vi "Measure vs B2DvsGatesweep.vi"() -> ()   [LabVIEW 2009]
doc: "This VI is an example operator panel.\n\nThe VI contains a table for the field values that may be configured manually, or loaded by checking the \"Prompt for File\" box. The data file should contain 3 columns of data, with each column delimited by a tab character.\n\nBefore the VI is executed, set the desired field units and coordinate system. Once the VI is started, follow the directions in the STATUS indicator to operate. Once a field value is achieved, it will be held indefinitely with no user intervention.\n\nThe present field is displayed in the selected units and coordinate system. The present field is queried once per second.\n\nIf a field point is specified that is outside the limits for the magnet, the VI will abort execution."
uses:
  <vilib>/Utility/file.llb/Read From Spreadsheet File (DBL).vi
panel:
  out "HP":T1(graph)={"measured data"=[130.77697934473076, 131.17238359064999, 131.57493282279165, 131.97089096284472, 132.3709005627829, 132.7747269835502, 133.17115299337118, 133.57699453159358, 133.97291907281786, 134.37163450772164, 134.7728190578919, 135.17563033959266, 135.57333372461295, 135.97830344291987, 136.37202071047088, 136.77617688548457, 137.17728611854096, 137.57344246367185, 137.96927398938195, 138.37484712631183, 138.7678966828463, 139.1744152195974, 139.5694101008014, 139.9620548045032, 140.3756352936819, 140.76443013035026, 141.1688823561444, 141.56815184223575, 141.9675976417151, 142.3659953584458, 142.775676716873, 143.16379154430956, 143.57809589273134, 143.96940395419173, 144.37063731617485, 144.76393855420042, 145.16100725100878, 145.5613313376955, 145.9608116195239, 146.37481274459287, 146.76791709360782, 147.16896149127172, 147.5663143604346, 147.9678028289989, 148.36962760092925, 148.76598884997566, 149.16767338072717, 149.56607764958403, 149.95999407346423, 150.3722468362733, 150.76361618206533, 151.15525055318153, 151.57358356130908, 151.9672547235955, 152.360163563412, 152.76137159791082, 153.15948892689605, 153.56793804327447, 153.9626908891637, 154.35791457944399, 154.76495537165297, 155.1633906497064, 155.56156935652382, 155.96111561211768, 156.36610319740612, 156.76559958179956, 157.17093878264262, 157.56689125105595, 157.96437052200662, 158.376205209266, 158.76161261329872, 159.16724590816438, 159.55971274891448, 159.96783078495864, 160.36059978391282, 160.75915896709176, 161.17541940848784, 161.56387349300712, 161.96414973052572, 162.36209894569686], "measured data"=[47.8127675, 47.3142275, 46.9315925, 46.6304225, 46.0396825, 45.6777125, 45.4570175, 45.070972499999996, 44.789265, 44.3558025, 43.6591325, 43.409885, 43.162465, 42.71473, 42.531679999999994, 42.226214999999996, 41.899212500000004, 41.3661625, 41.03545, 40.637135, 40.367885, 40.046705, 39.865300000000005, 39.57427, 39.035422499999996, 38.758669999999995, 38.5814575, 38.362825, 37.764005, 37.63395250000001, 37.1175925, 15.572479999999999, -4.558832499999999, -4.02452, 18.98894, -4.1475925, -5.032675, 25.0248675, 27.1825925, 28.551062500000004, 27.772665, 26.5350725, 23.5985575, 27.104, 24.8567975, 23.797494999999998, 25.486569999999997, 24.9155175, 26.26794, 24.482997499999996, 25.039457499999997, 13.34384, 13.3442075, 13.3447275, 13.34462, 13.344155, 54.256817500000004, 13.3434, 13.3445175, 13.343632500000002, 13.3429575, 13.343734999999999, 13.3441525, -7.896862499999999, 13.344205, -8.8820475, 13.343815, 13.3419875, -24.604432499999998, 13.342722499999999, -6.686962499999998, 13.34337, 13.343815, 13.344335000000001, -23.786430000000003, 13.34392, 13.343657499999999, 13.3431125, 13.3426425, 13.342744999999999]}
  in  "go to zero at end of measurement":bool=TRUE
  out "fieldvalues":string[](array[string])=["0.5", "91"]
  out "LI":T1(graph)={"measured data"=[130.77697934473076, 131.17238359064999, 131.57493282279165, 131.97089096284472, 132.3709005627829, 132.7747269835502, 133.17115299337118, 133.57699453159358, 133.97291907281786, 134.37163450772164, 134.7728190578919, 135.17563033959266, 135.57333372461295, 135.97830344291987, 136.37202071047088, 136.77617688548457, 137.17728611854096, 137.57344246367185, 137.96927398938195, 138.37484712631183, 138.7678966828463, 139.1744152195974, 139.5694101008014, 139.9620548045032, 140.3756352936819, 140.76443013035026, 141.1688823561444, 141.56815184223575, 141.9675976417151, 142.3659953584458, 142.775676716873, 143.16379154430956, 143.57809589273134, 143.96940395419173, 144.37063731617485, 144.76393855420042, 145.16100725100878, 145.5613313376955, 145.9608116195239, 146.37481274459287, 146.76791709360782, 147.16896149127172, 147.5663143604346, 147.9678028289989, 148.36962760092925, 148.76598884997566, 149.16767338072717, 149.56607764958403, 149.95999407346423, 150.3722468362733, 150.76361618206533, 151.15525055318153, 151.57358356130908, 151.9672547235955, 152.360163563412, 152.76137159791082, 153.15948892689605, 153.56793804327447, 153.9626908891637, 154.35791457944399, 154.76495537165297, 155.1633906497064, 155.56156935652382, 155.96111561211768, 156.36610319740612, 156.76559958179956, 157.17093878264262, 157.56689125105595, 157.96437052200662, 158.376205209266, 158.76161261329872, 159.16724590816438, 159.55971274891448, 159.96783078495864, 160.36059978391282, 160.75915896709176, 161.17541940848784, 161.56387349300712, 161.96414973052572, 162.36209894569686], "measured data"=[47.8127675, 47.3142275, 46.9315925, 46.6304225, 46.0396825, 45.6777125, 45.4570175, 45.070972499999996, 44.789265, 44.3558025, 43.6591325, 43.409885, 43.162465, 42.71473, 42.531679999999994, 42.226214999999996, 41.899212500000004, 41.3661625, 41.03545, 40.637135, 40.367885, 40.046705, 39.865300000000005, 39.57427, 39.035422499999996, 38.758669999999995, 38.5814575, 38.362825, 37.764005, 37.63395250000001, 37.1175925, 15.572479999999999, -4.558832499999999, -4.02452, 18.98894, -4.1475925, -5.032675, 25.0248675, 27.1825925, 28.551062500000004, 27.772665, 26.5350725, 23.5985575, 27.104, 24.8567975, 23.797494999999998, 25.486569999999997, 24.9155175, 26.26794, 24.482997499999996, 25.039457499999997, 13.34384, 13.3442075, 13.3447275, 13.34462, 13.344155, 54.256817500000004, 13.3434, 13.3445175, 13.343632500000002, 13.3429575, 13.343734999999999, 13.3441525, -7.896862499999999, 13.344205, -8.8820475, 13.343815, 13.3419875, -24.604432499999998, 13.342722499999999, -6.686962499999998, 13.34337, 13.343815, 13.344335000000001, -23.786430000000003, 13.34392, 13.343657499999999, 13.3431125, 13.3426425, 13.342744999999999]}
  in  "Wait between \nVectors":bool=TRUE
  in  "PID Off":bool
  in  "Wait between \nVectors (ms)":u32=4000
  out "measured data":dbl[][](array[numeric])
  in  "Notes:":string="Datum: 6.04.12, Uhrzeit: 12:30,  T 4K,Winkelsweep 1° Winkelschritte, warten bei jedem Feldpunkt (measurevsB2Dv9.vi))4s, vectorsm1.txt, praktikumsprobenstab, Sweep  0.15, CrB auf CuBe Sensoren" caption="Notizen:"
  in  "Measurement File":path=path "D:/UserData/Matthias/Messungen/STO_LAOR124aufCantilever/120523/120523_R124_Gatevst"
  in  "Sample name:":string="CrB"
  in  "HP 1":bool=TRUE
  in  "GPIB HP":string="13"
  in  "LI 1":bool
  in  "GPIB L 1":string="8"
  out "Number of lines":i32=2
  in  "Operation":u16(ring)=1 items=["Stepwise", "Continous"]
  out "Ramp Rate along Vector (T/min)":dbl=0.15 format="%.3f"
  out "Current Ramp Rate Z (T/min)":dbl=0.015702717677741673 format="%.3f"
  out "Current Ramp Rate Y (T/min)":dbl=0.1491758179382072 format="%.3f"
  in  "User defined Ramp Rate (T/min)":bool=TRUE
  in  "User defined Ramp Rate (T/min)":dbl=0.5 format="%.3f"
  in  "Z-Axis Communications Config":T2={"GPIB address"=22, "GPIB bus"=1, "connection ID"=refnum, "IP"="111.111.111.1", "Active Comm Interface"=0, "Serial Port"="", "Programmer Type"=0} {"Programmer Type" items=["Model 430", "Model 420"]; "Active Comm Interface" items=["TCP/IP (Model 430 Only)", "RS232", "IEEE488"]}
  in  "Max Ramp Rate - Y Axis (A/s)":dbl=0.055 format="%.3f"
  in  "Max Ramp Rate - Z Axis (A/s)":dbl=0.19 format="%.3f"
  in  "Magnitude Limit (kG)":dbl=45.1 format="%.3f"
  in  "Y-Axis Communications Config":T2={"GPIB address"=22, "GPIB bus"=1, "connection ID"=refnum, "IP"="111.111.111.2", "Active Comm Interface"=0, "Serial Port"="", "Programmer Type"=0} {"Programmer Type" items=["Model 430", "Model 420"]; "Active Comm Interface" items=["TCP/IP (Model 430 Only)", "RS232", "IEEE488"]}
  out "Cartesian Display (T)":T3={"Y-Axis Field (T)"=0.01746, "Z-Axis Field (T)"=0.99986} {"Z-Axis Field (T)" format="%.3f"; "Y-Axis Field (T)" format="%.3f"}
  in  "Starting index":i32=1
  in  "Normal color":u32(colorbox)=11711154
  in  "Highlight color":u32(colorbox)=16711680
  in  "Prompt for File?":bool
  out "Continue Execution?":bool=TRUE
  out "error out":T4
  in  "error in":T4
  out "STATUS":string="Ramping to field vector 1..."
  in  "Ramping Control":u16(ring)=1 items=["NEXT VECTOR", "RAMPING", "HOLDING", "PAUSE", "ZERO"]
  out "Cartesian Display (kG)":T5 {"Z-Axis Field (kG)" format="%.3f"; "Y-Axis Field (kG)" format="%.3f"}
  in  "Field Values":string[][](table)=[["0", "1"], ["0", "0.5"]]
  out "Switch Heaters":bool=TRUE
  out "Polar Display (T)":T6={"q (degrees)"=89.97708168941708, "Field Magnitude (T)"=0.5000000399999984} {"Field Magnitude (T)" format="%.3f"; "q (degrees)" format="%.3f"}
  out "Polar Display (kG)":T7 {"Field Magnitude (kG)" format="%.3f"; "q (degrees)" format="%.3f"}
  in  "Coordinate System":u16(ring) items=["Cartesian", "Polar"]
  in  "Magnetic Field Units":u16(ring)=1 items=["kG", "Tesla"]
  # "Punkt für Punkt Messung, gotozero am Ende der Messung und switch heater off"
  # "Measurement Display"
  # "Measurement Settings"
  # "Magnet Settings"
  # "Max Ramp Rate z: 1.27 T/min\nMax Ramp Rate y: 0.17 T/min"
  # "Devices"
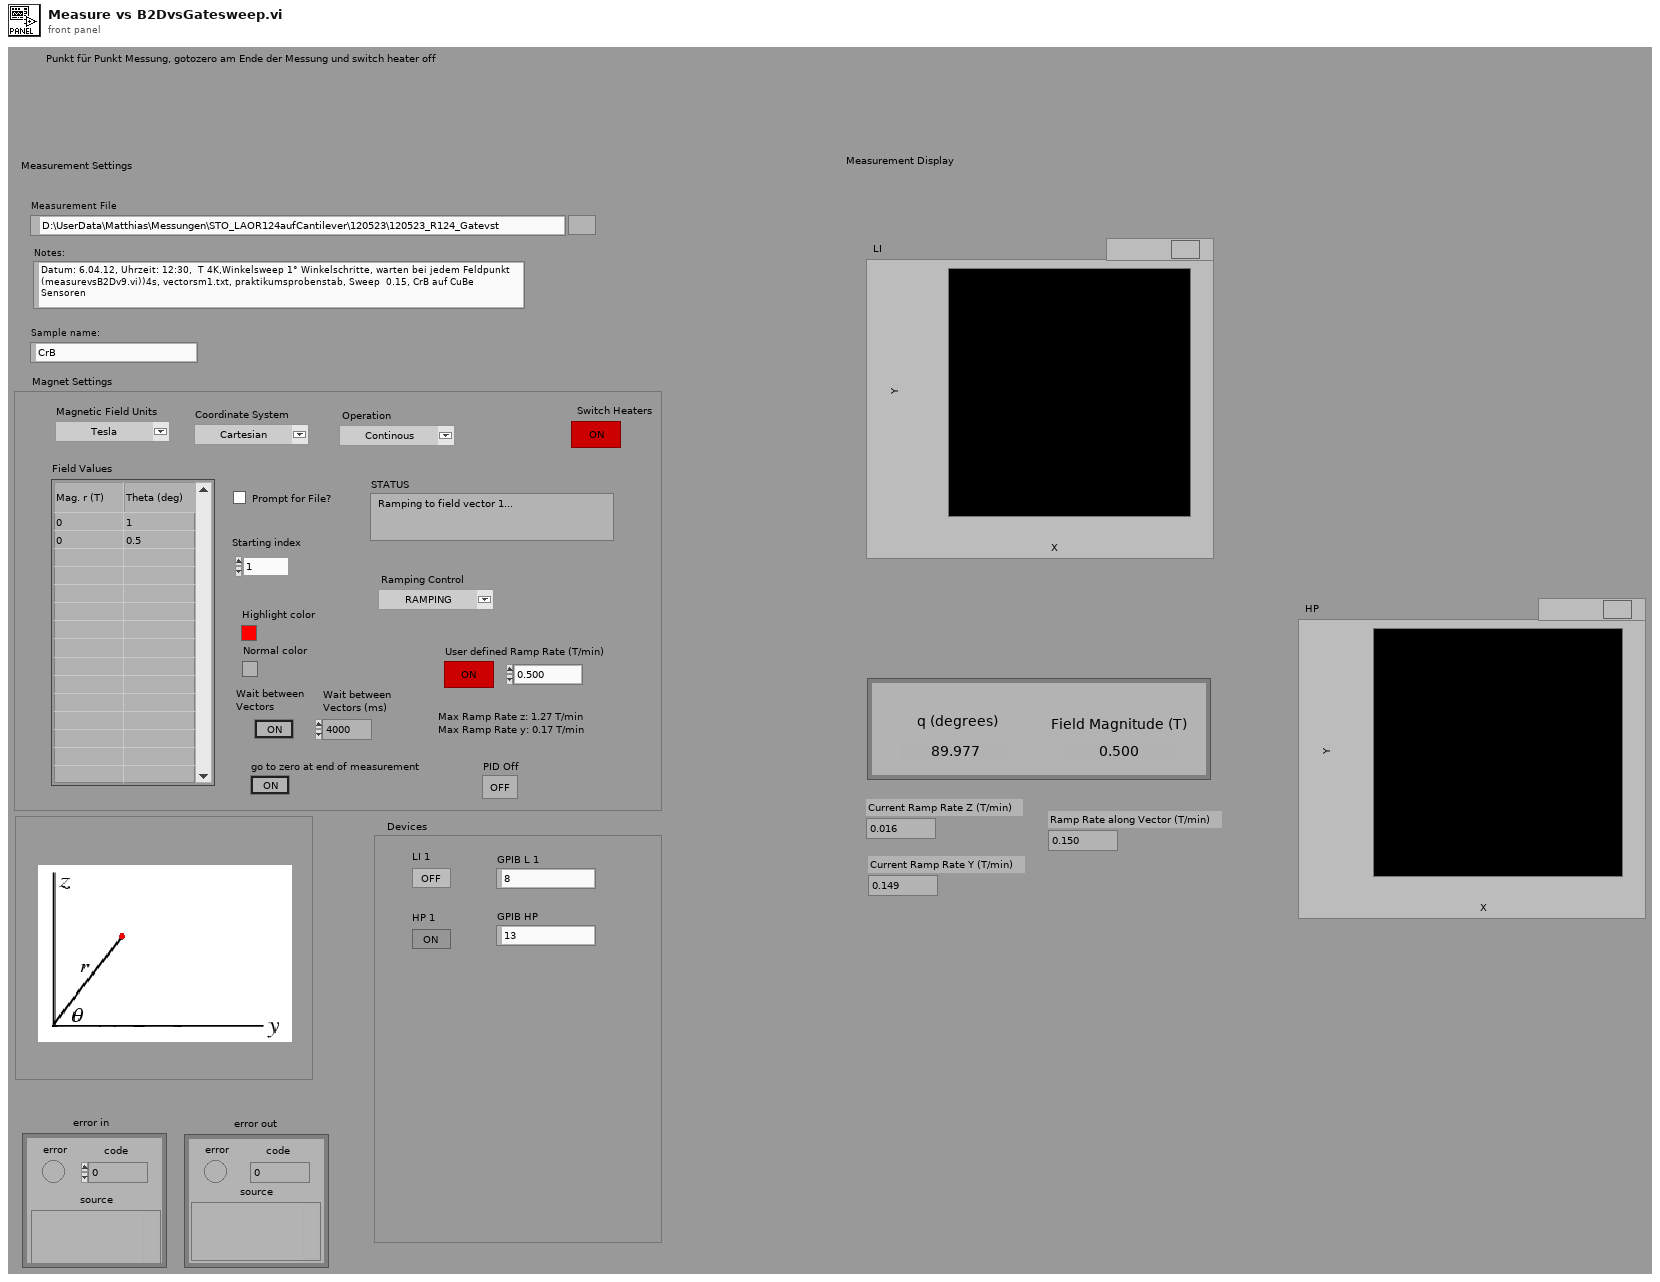
[diagram p1: front panel]
types:
  T1 = cluster{"measured data":dbl[], "measured data":dbl[]}
  T2 = cluster{"GPIB address":i16, "GPIB bus":i16, "connection ID":refnum<k5>, "IP":string, "Active Comm Interface":u16, "Serial Port":refnum<visa-resource-name>, "Programmer Type":u16}
  T3 = cluster{"Y-Axis Field (T)":dbl, "Z-Axis Field (T)":dbl}
  T4 = cluster{"error":bool, "code":i32, "source":string}
  T5 = cluster{"Y-Axis Field (kG)":dbl, "Z-Axis Field (kG)":dbl}
  T6 = cluster{"q (degrees)":dbl, "Field Magnitude (T)":dbl}
  T7 = cluster{"q (degrees)":dbl, "Field Magnitude (kG)":dbl}
  T8 = enum16{"", "RAMPING", "HOLDING", "PAUSED", "MANUAL UP", "MANUAL DOWN", "ZEROING CURRENT", "QUENCH DETECTED", "HEATING SWITCH"}
  T9 = enum16{"", "RAMPING", "HOLDING", "PAUSED", "MANUAL UP", "MANUAL DOWN", "ZEROING CURRENT", "QUENCH DETECTED", "HEATING SWITCH", "AT ZER0", "COOLING SWITCH"}
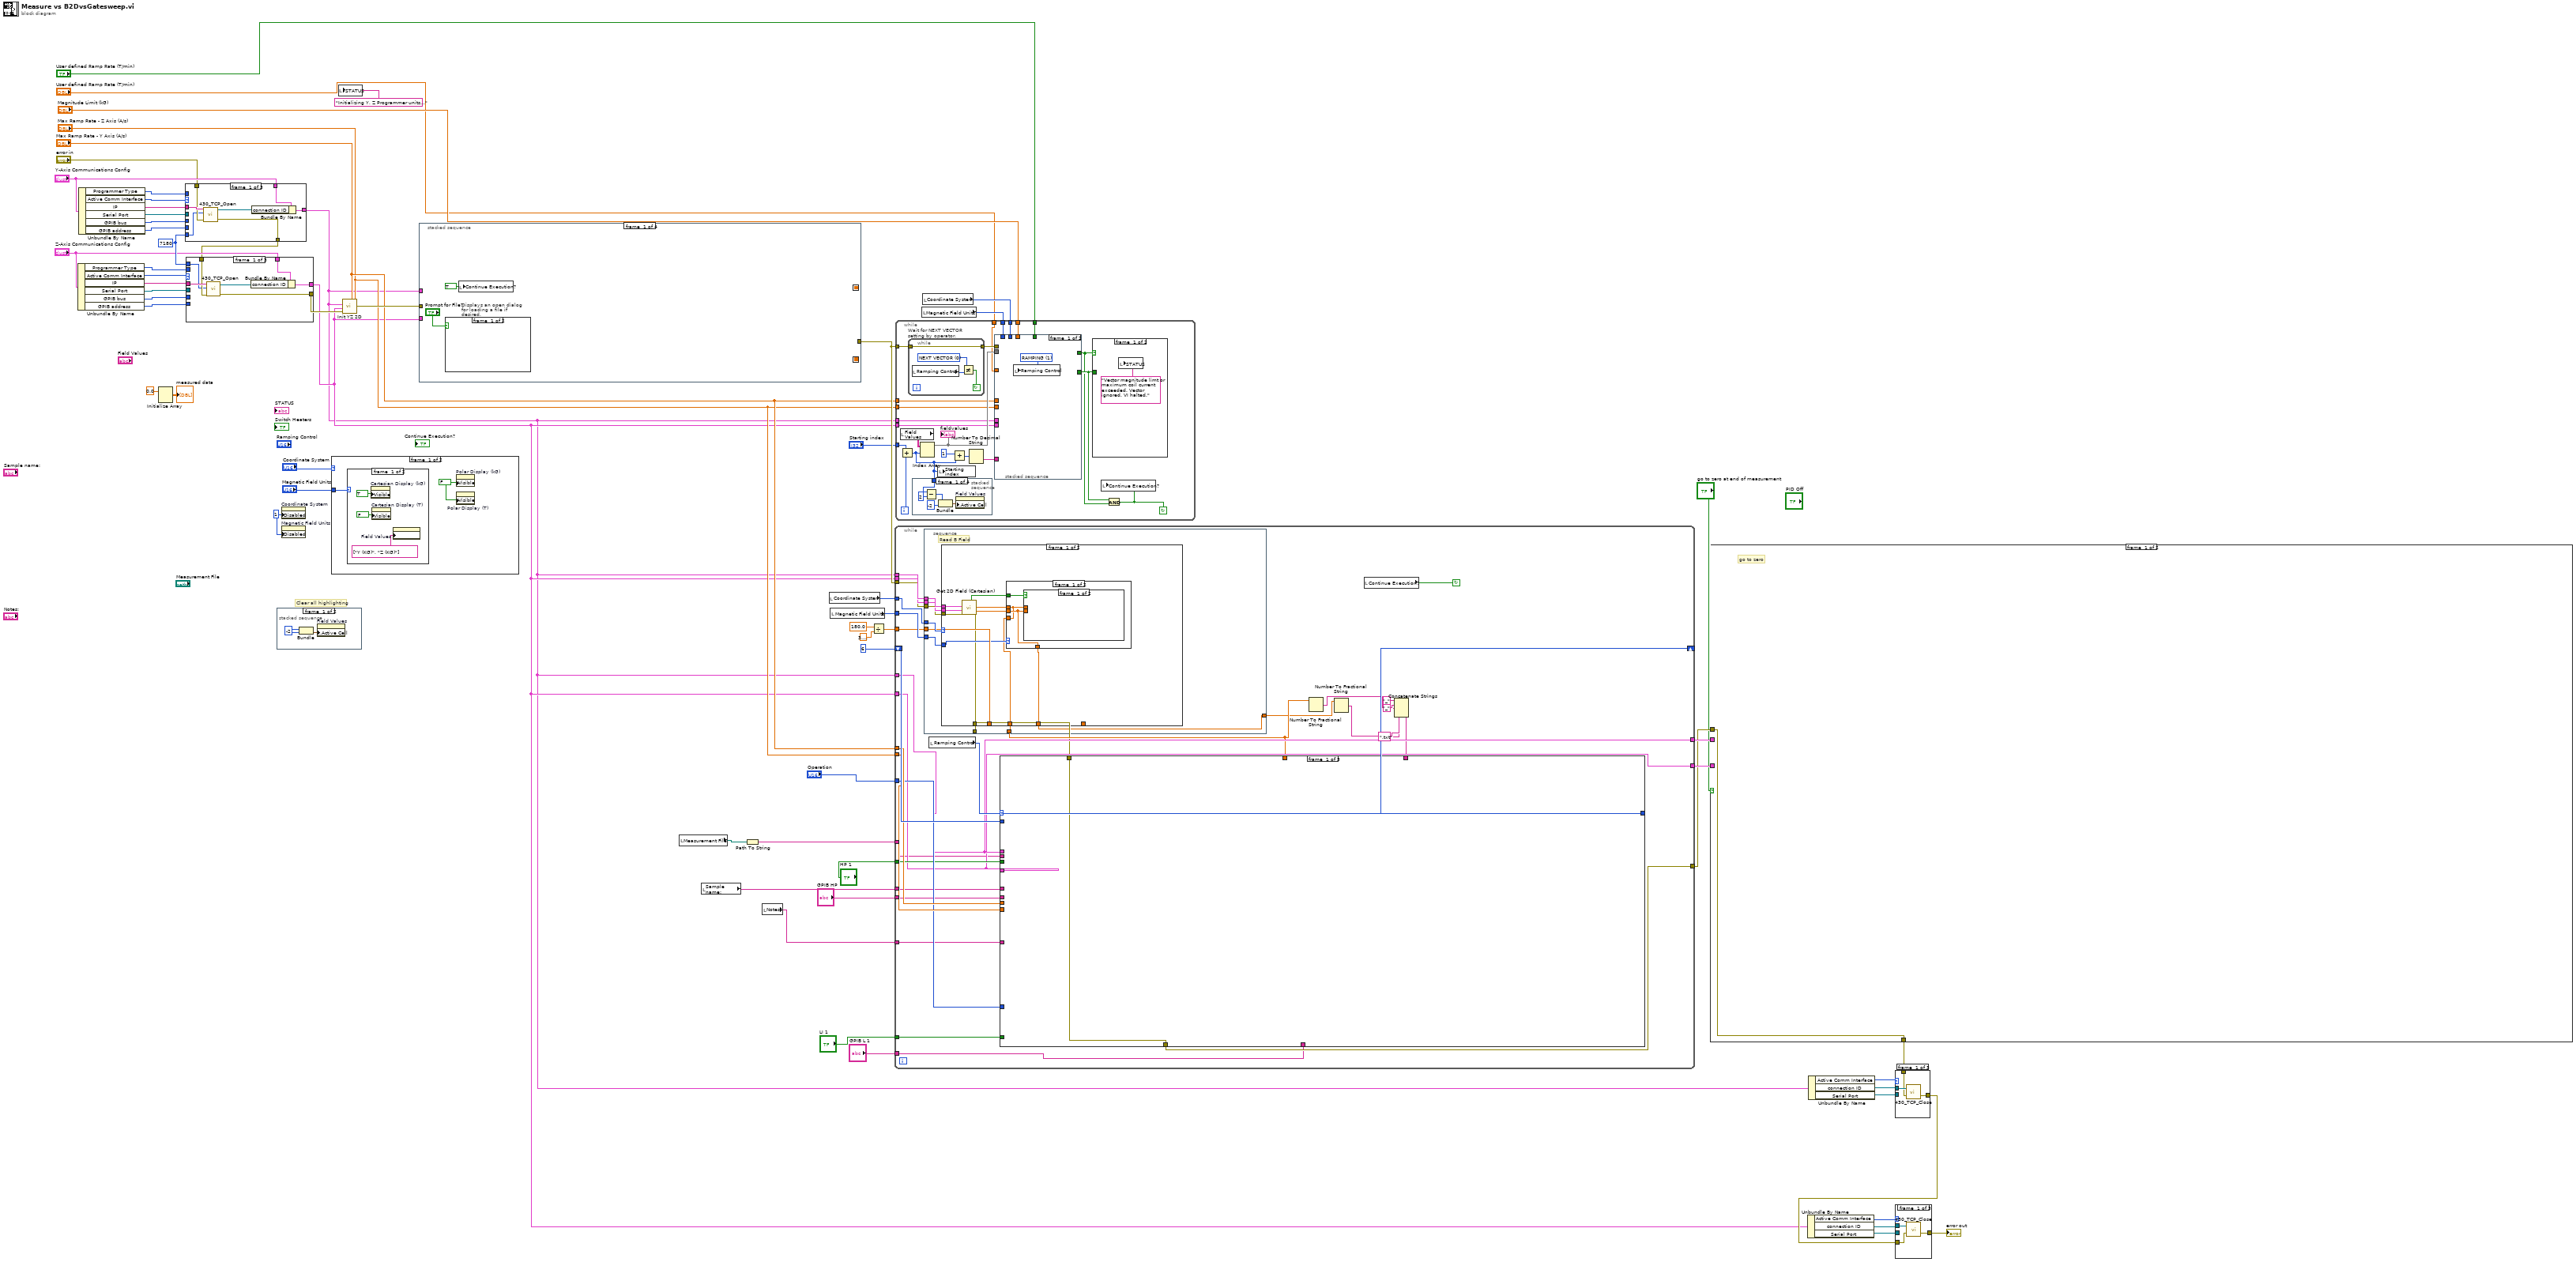
[diagram p0: block diagram]
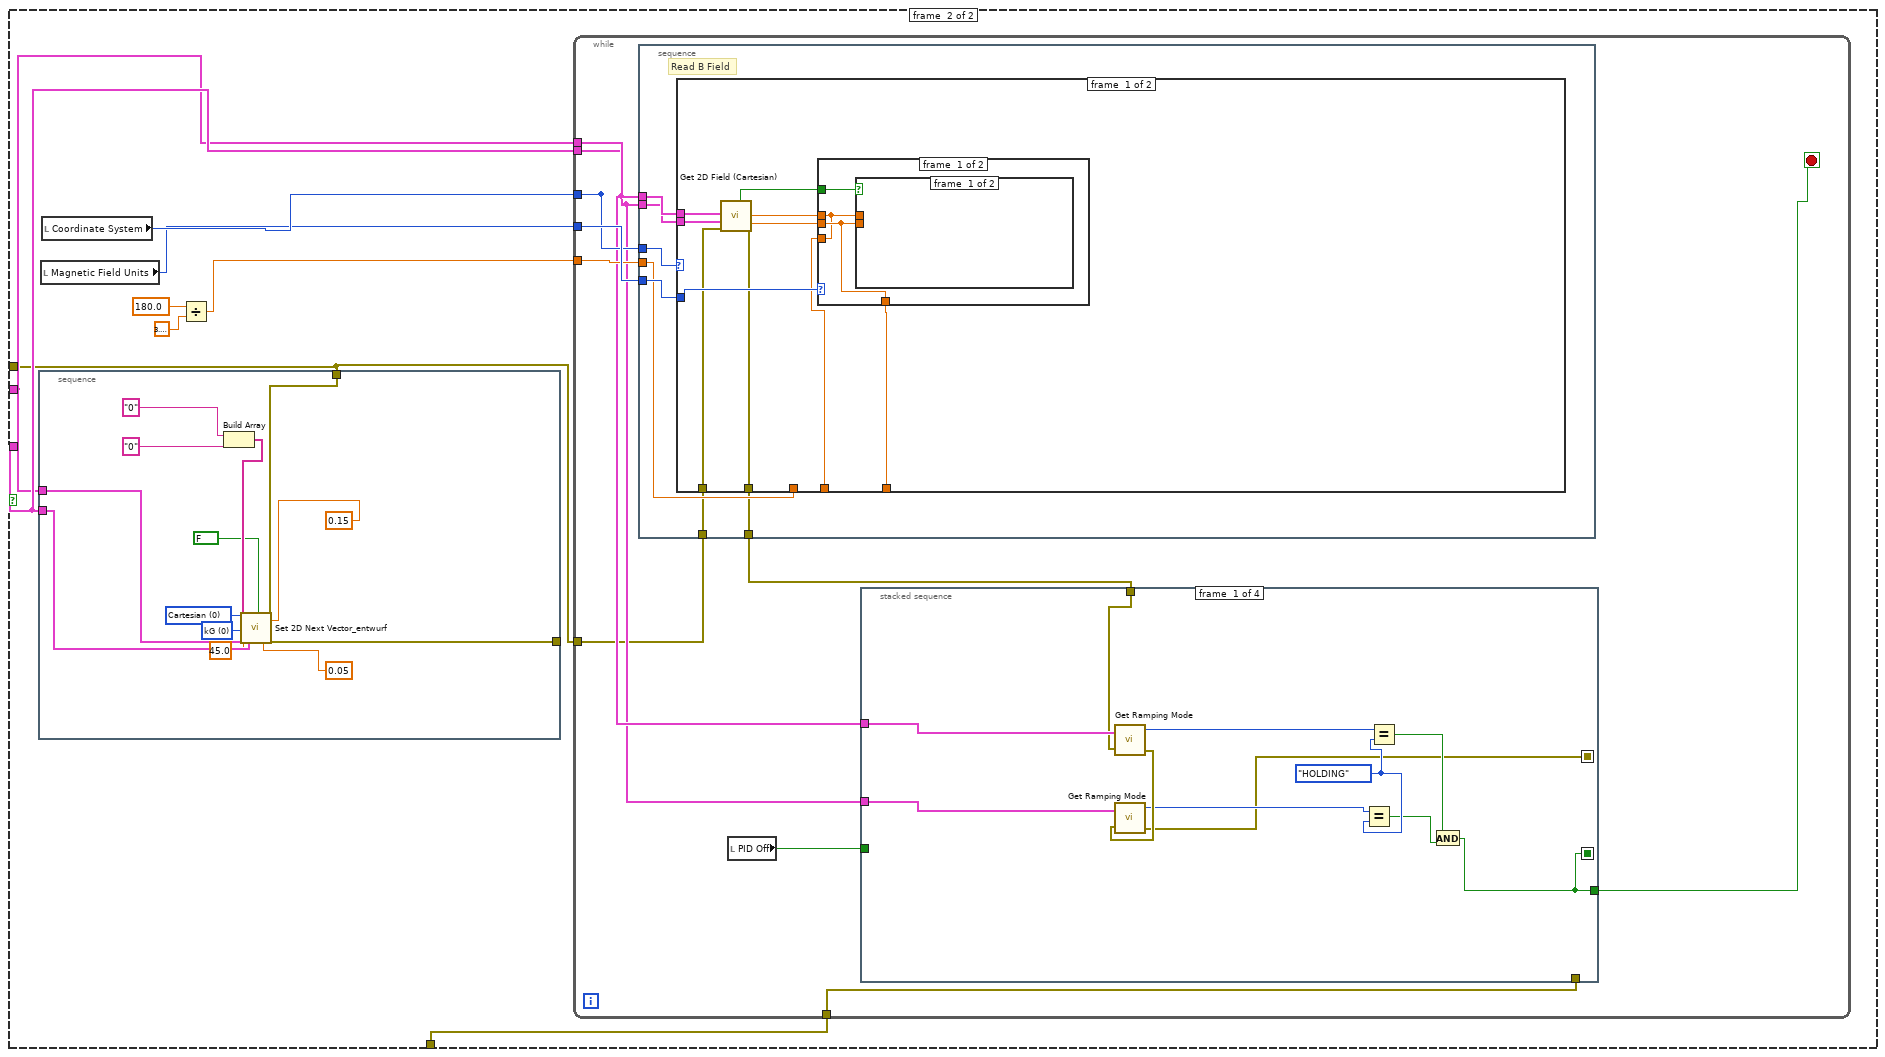
[diagram p2: hidden frame]
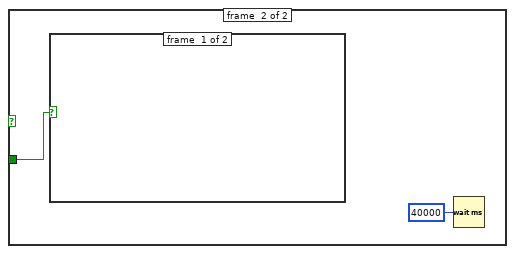
[diagram p4: hidden frame]
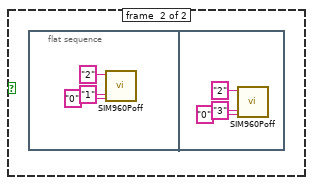
[diagram p5: hidden frame]
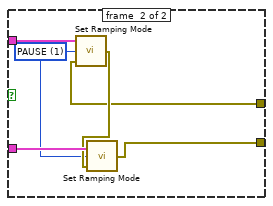
[diagram p7: hidden frame]
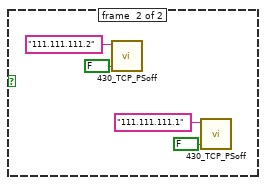
[diagram p9: hidden frame]
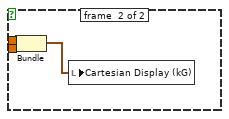
[diagram p10: hidden frame]
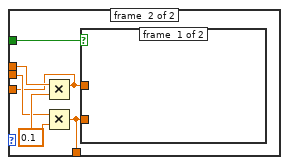
[diagram p11: hidden frame]
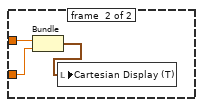
[diagram p12: hidden frame]
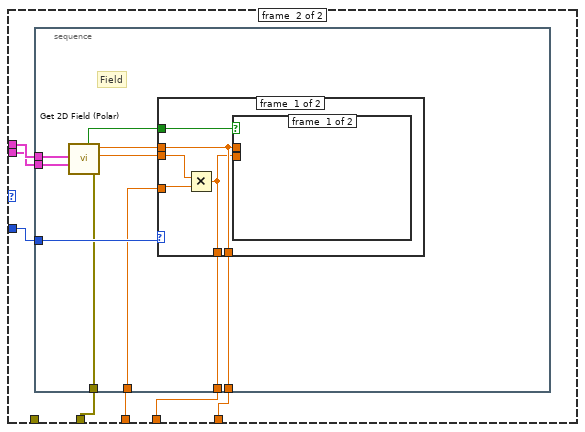
[diagram p13: hidden frame]
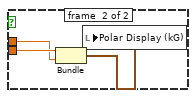
[diagram p14: hidden frame]
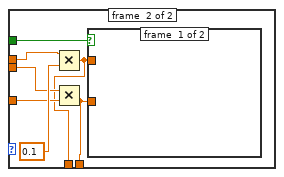
[diagram p15: hidden frame]
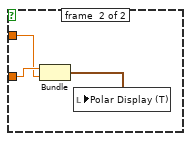
[diagram p16: hidden frame]
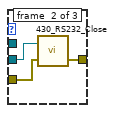
[diagram p17: hidden frame]
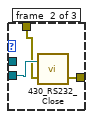
[diagram p19: hidden frame]
diagram:
  w49 = 7180 ("TCP Port")
  w62 = u8 1 ("Write Attribute")
  # "Clear all highlighting"
  n1 = Unbundle By Name("Z-Axis Communications Config") -> ("Programmer Type"=w28:u16, "Active Comm Interface"=w48:u16, "IP"=w45:string, "Serial Port"=w44:refnum<visa-resource-name>, "GPIB bus"=w27:i16, "GPIB address"=w26:i16)
  n2 = Unbundle By Name("Y-Axis Communications Config") -> ("Programmer Type"=w22:u16, "Active Comm Interface"=w47:u16, "IP"=w46:string, "Serial Port"=w43:refnum<visa-resource-name>, "GPIB bus"=w23:i16, "GPIB address"=w24:i16)
  n3 = Initialize Array(0.0 ("element")) -> (→"measured data":dbl[][])  [unwired: 2 in]
  n4 = case shown="2" w47 {
    tunnel: w46 -> [w71 _ _]
    tunnel: "error in" -> [w70 w77 w79]
    tunnel: "Y-Axis Communications Config" -> [w69 w72 w83]
    tunnel: [w67 w75 w83] -> w11
    tunnel: [w66 w76 w78] -> w25
    tunnel: w49 -> [w65 _ _]
    tunnel: w43 -> [_ w73 _]
    tunnel: w24 -> [_ _ w82]
    tunnel: w23 -> [_ _ w81]
    tunnel: w22 -> [_ _ w80]
    frame #0 {
      n5 = call <userlib>:"430_TCP_Open.vi"("IP Address"=w71, "TCP Port"=w65, "error in (no error)"=w70) -> ("connection ID"=w68:refnum<k5>, "error out"=w66:errorcluster)  [unwired: 3 in, 1 out]
      n6 = Bundle By Name(cluster=w69, "connection ID"=w68) -> (w67:T2)
    }
    frame #1 {
      n7 = call <userlib>:"430_RS232_Open.vi"("VISA resource name"=w73, "error in (no error)"=w77) -> ("VISA resource name out"=w74:refnum<visa-resource-name>, "error out"=w76:errorcluster)  [unwired: 5 in]
      n8 = Bundle By Name(cluster=w72, "Serial Port"=w74) -> (w75:T2)
    }
    frame #2 {
      n9 = case shown="0, Default" w80 {
        tunnel: w81 -> [w87 _]
        tunnel: w82 -> [w86 _]
        tunnel: w79 -> [w85 w88]
        tunnel: [w84 w88] -> w78
        frame #0 {
          n10 = DevClear(2:w85, 3:w86, 4:w87) -> (0:w84:errorcluster)  [unwired: 1 out]
        }
        frame #1 {
        }
      }
    }
  }
  n11 = case shown="2" w48 {
    tunnel: w45 -> [w95 _ _]
    tunnel: w25 -> [w94 w101 w103]
    tunnel: [w93 w100 w102] -> w42
    tunnel: "Z-Axis Communications Config" -> [w92 w98 w107]
    tunnel: [w90 w99 w107] -> w12
    tunnel: w49 -> [w89 _ _]
    tunnel: w44 -> [_ w96 _]
    tunnel: w28 -> [_ _ w106]
    tunnel: w27 -> [_ _ w105]
    tunnel: w26 -> [_ _ w104]
    frame #0 {
      n12 = call <userlib>:"430_TCP_Open.vi"("IP Address"=w95, "TCP Port"=w89, "error in (no error)"=w94) -> ("connection ID"=w91:refnum<k5>, "error out"=w93:errorcluster)  [unwired: 3 in, 1 out]
      n13 = Bundle By Name(cluster=w92, "connection ID"=w91) -> (w90:T2)
    }
    frame #1 {
      n14 = call <userlib>:"430_RS232_Open.vi"("VISA resource name"=w96, "error in (no error)"=w101) -> ("VISA resource name out"=w97:refnum<visa-resource-name>, "error out"=w100:errorcluster)  [unwired: 5 in]
      n15 = Bundle By Name(cluster=w98, "Serial Port"=w97) -> (w99:T2)
    }
    frame #2 {
      n16 = case shown="0, Default" w106 {
        tunnel: w105 -> [w111 _]
        tunnel: w104 -> [w110 _]
        tunnel: w103 -> [w109 w112]
        tunnel: [w108 w112] -> w102
        frame #0 {
          n17 = DevClear(2:w109, 3:w110, 4:w111) -> (0:w108:errorcluster)  [unwired: 1 out]
        }
        frame #1 {
        }
      }
    }
  }
  n18 = stacked-sequence {
    frame #0 {
      w113 = -2
      n19 = Bundle(w113, w113) -> (w114:cluster{i32, i32})  [unwired: 1 in]
      n20 = property on="Field Values" class="Tbl (strict)"("Active Cell:Active Cell"=w114) -> ()  [unwired: 2 in, 2 out]
    }
    frame #1 {
      n21 = property on="Field Values" class="Tbl (strict)"("Active Cell:Cell Background Color"="Normal color") -> ()  [unwired: 2 in, 2 out]
    }
  }
  n22 = property on="Coordinate System" class="Ring (strict)"("Disabled"=w62) -> ()  [unwired: 2 in, 2 out]
  n23 = property on="Magnetic Field Units" class="Ring (strict)"("Disabled"=w62) -> ()  [unwired: 2 in, 2 out]
  n24 = case shown="0, Default" "Coordinate System" {
    tunnel: "Magnetic Field Units" -> [w117 w125]
    frame #0 {
      w116 = FALSE ("Write Attribute")
      (unwired) FALSE ("Write Attribute")
      (unwired) TRUE ("Write Attribute")
      n25 = case shown="1" w117 {
        frame #0 {
          n26 = property on="Cartesian Display (kG)" class="Cluster (strict)"("Visible"=TRUE ("Write Attribute")) -> ()  [unwired: 2 in, 2 out]
          n27 = property on="Cartesian Display (T)" class="Cluster (strict)"("Visible"=FALSE ("Write Attribute")) -> ()  [unwired: 2 in, 2 out]
          n28 = property on="Field Values" class="Tbl (strict)"("Column Header Strings[]"=string[] ["Y (KG)", "Z (KG)"] ("Write Attribute")) -> ()  [unwired: 2 in, 2 out]
        }
        frame #1 {
          n29 = property on="Cartesian Display (kG)" class="Cluster (strict)"("Visible"=FALSE ("Write Attribute")) -> ()  [unwired: 2 in, 2 out]
          n30 = property on="Cartesian Display (T)" class="Cluster (strict)"("Visible"=TRUE ("Write Attribute")) -> ()  [unwired: 2 in, 2 out]
          n31 = property on="Field Values" class="Tbl (strict)"("Column Header Strings[]"=string[] ["Y (T)", "Z (T)"] ("Write Attribute")) -> ()  [unwired: 2 in, 2 out]
        }
      }
      n32 = property on="Polar Display (kG)" class="Clust (strict)"("Visible"=w116) -> ()  [unwired: 2 in, 2 out]
      n33 = property on="Polar Display (T)" class="Clust (strict)"("Visible"=w116) -> ()  [unwired: 2 in, 2 out]
    }
    frame #1 {
      (unwired) FALSE ("Write Attribute")
      (unwired) TRUE ("Write Attribute")
      w124 = FALSE ("Write Attribute")
      n34 = case shown="1" w125 {
        frame #0 {
          n35 = property on="Polar Display (kG)" class="Clust (strict)"("Visible"=TRUE ("Write Attribute")) -> ()  [unwired: 2 in, 2 out]
          n36 = property on="Polar Display (T)" class="Clust (strict)"("Visible"=FALSE ("Write Attribute")) -> ()  [unwired: 2 in, 2 out]
          n37 = property on="Field Values" class="Tbl (strict)"("Column Header Strings[]"=string[] ["Mag. r (KG)", "Theta (deg)"] ("Write Attribute")) -> ()  [unwired: 2 in, 2 out]
        }
        frame #1 {
          n38 = property on="Polar Display (kG)" class="Clust (strict)"("Visible"=FALSE ("Write Attribute")) -> ()  [unwired: 2 in, 2 out]
          n39 = property on="Polar Display (T)" class="Clust (strict)"("Visible"=TRUE ("Write Attribute")) -> ()  [unwired: 2 in, 2 out]
          n40 = property on="Field Values" class="Tbl (strict)"("Column Header Strings[]"=string[] ["Mag. r (T)", "Theta (deg)"] ("Write Attribute")) -> ()  [unwired: 2 in, 2 out]
        }
      }
      n41 = property on="Cartesian Display (kG)" class="Cluster (strict)"("Visible"=w124) -> ()  [unwired: 2 in, 2 out]
      n42 = property on="Cartesian Display (T)" class="Cluster (strict)"("Visible"=w124) -> ()  [unwired: 2 in, 2 out]
    }
  }
  n43 = local write "STATUS"("Initializing Y, Z Programmer units..." ("STATUS")) -> ()
  n44 = call <userlib>:"Init YZ 2D.vi"("Max Ramp Rate Z-axis"="Max Ramp Rate - Z Axis (A/s)", "Max Ramp Rate Y-axis"="Max Ramp Rate - Y Axis (A/s)", "error in"=w42, "Z-Axis Communications Config"=w12, "Y-Axis Communications Config"=w11) -> ("error out"=w60:T4)  [unwired: 5 in]
  n45 = stacked-sequence {
    seq-local: [_ w139 _ _] -> [_ _ w186 _]
    seq-local: [_ w138 _ _] -> [_ _ w185 _]
    tunnel: w12 -> [_ w141 _ _]
    tunnel: w60 -> [_ w142 _ _]
    tunnel: [_ w137 _ _] -> w56
    tunnel: w11 -> [_ w140 _ _]
    frame #0 {
      n46 = case "Displays an open dialog for loading a file if desired." shown="True" "Prompt for File?" {
        frame #0 {
        }
        frame #1 {
          n47 = call-poly <vilib>:"Read From Spreadsheet File.vi"() -> ("all rows"=w136:dbl[][])  [unwired: 7 in, 4 out]
          n48 = Number To Fractional String(number=w136, precision (6)=i16 4) -> (F-format string=w135:string[][])  [unwired: 2 in]
          n49 = local write "Field Values"(w135) -> ()
        }
      }
      n50 = local write "Continue Execution?"(TRUE ("Continue Execution?")) -> ()
    }
    frame #1 {
      w150 = u16 3 items=["NEXT VECTOR", "RAMPING", "HOLDING", "PAUSE", "ZERO"] ("Ramping Control")
      n51 = call <userlib>:"Get Switch Present.vi"("error in"=w142, "Communications Config"=w140) -> ("error out"=w146:T4, "Switch Present?"=w147:bool)
      n52 = case shown="True" w147 {
        tunnel: w146 -> [w168 w177]
        tunnel: w140 -> [_ w170]
        tunnel: [0.0 w174] -> w138
        tunnel: [w168 w176] -> w145
        frame #0 {
        }
        frame #1 {
          n53 = call <userlib>:"Get Switch Heater Time.vi"("error in"=w177, "Communications Config"=w170) -> ("error out"=w173:T4, "Switch Heating Time (secs)"=w175:dbl)
          n54 = call <userlib>:"Get Switch Heater.vi"("error in"=w173, "Communications Config"=w170) -> ("error out"=w172:T4, "Switch Heater Indicator"=w171:bool)
          n55 = case shown="False" w171 {
            tunnel: [w182 w183] -> w176
            tunnel: w175 -> [w180 _]
            tunnel: [w180 0.0] -> w174
            tunnel: w172 -> [w178 w183]
            tunnel: w170 -> [w179 _]
            frame #0 {
              n56 = call <userlib>:"Set Switch Heater.vi"("error in"=w178, "Switch Heater Control"=TRUE, "Communications Config"=w179) -> ("error out"=w182:T4)
            }
            frame #1 {
            }
          }
        }
      }
      n57 = call <userlib>:"Get Switch Present.vi"("error in"=w145, "Communications Config"=w141) -> ("error out"=w143:T4, "Switch Present?"=w144:bool)
      n58 = case shown="True" w144 {
        tunnel: w143 -> [w151 w160]
        tunnel: w141 -> [_ w153]
        tunnel: [0.0 w157] -> w139
        tunnel: [w151 w159] -> w137
        frame #0 {
        }
        frame #1 {
          n59 = call <userlib>:"Get Switch Heater Time.vi"("error in"=w160, "Communications Config"=w153) -> ("error out"=w156:T4, "Switch Heating Time (secs)"=w158:dbl)
          n60 = call <userlib>:"Get Switch Heater.vi"("error in"=w156, "Communications Config"=w153) -> ("error out"=w155:T4, "Switch Heater Indicator"=w154:bool)
          n61 = case shown="False" w154 {
            tunnel: [w161 w166] -> w159
            tunnel: w158 -> [w164 _]
            tunnel: [w164 0.0] -> w157
            tunnel: w155 -> [w162 w166]
            tunnel: w153 -> [w163 _]
            frame #0 {
              n62 = call <userlib>:"Set Switch Heater.vi"("error in"=w162, "Switch Heater Control"=TRUE, "Communications Config"=w163) -> ("error out"=w161:T4)
            }
            frame #1 {
            }
          }
        }
      }
      n63 = local write "Ramping Control"(w150) -> ()
      n64 = local write "Switch Heaters"(TRUE ("Switch Heater Control")) -> ()
      n65 = property on="Switch Heaters" class="Boolean (strict)"("Disabled"=u8 1 ("Write Attribute")) -> ()  [unwired: 2 in, 2 out]
    }
    frame #2 {
      n66 = Max & Min(x=w186, y=w185) -> (max(x,y)=w187:dbl)  [unwired: 1 out]
      n67 = local write "STATUS"("Heating switches..." ("STATUS")) -> ()
      n68 = Add(x=w187, y=2) -> (x+y=w191:dbl)
      n69 = property on="Ramping Control" class="Ring (strict)"("Disabled"=u8 1 ("Write Attribute")) -> ()  [unwired: 2 in, 2 out]
      n70 = Multiply(x=w191, y=1000) -> (x*y=w190:dbl)
      n71 = Wait (ms)(milliseconds to wait=w190) -> ()  [unwired: 1 out]
    }
    frame #3 {
      n72 = property on="Ramping Control" class="Ring (strict)"("Disabled"=u8 0 ("Write Attribute")) -> ()  [unwired: 2 in, 2 out]
      n73 = local write "STATUS"("Ready to ramp to first vector. Set Ramping Mode to NEXT VECTOR to begin." ("STATUS")) -> ()
      n74 = local read "Field Values"() -> (w196:string[][])
      n75 = Array Size(array=w196) -> (size(s)=w195:i32[])
      n76 = Index Array(array=w195, index=0) -> (element=→"Number of lines":i32)
    }
  }
  n77 = local read "Measurement File"() -> (w2:path)
  n78 = local read "Sample name:"() -> (w3:string)
  n79 = Path To String(path=w2) -> (string=w1:string)
  n80 = local read "Notes:"() -> (w4:string)
  n81 = local read "Coordinate System"() -> (w57:u16)
  n82 = local read "Magnetic Field Units"() -> (w55:u16)
  n83 = Divide(x=180.0, y=3.141592653589793) -> (x/y=w52:dbl)
  n84 = while {
    shift-left: u16 6 ("Ramping Control") -> [w222]
    shift-right: [w223] -> _
    tunnel: [w225] -> w7
    tunnel: w12 -> [w212]
    tunnel: w11 -> [w213]
    tunnel: w52 -> [w227]
    tunnel: w55 -> [w228]
    tunnel: w56 -> [w229]
    tunnel: w12 -> [w230]
    tunnel: w11 -> [w231]
    tunnel: w57 -> [w218]
    tunnel: "Max Ramp Rate - Y Axis (A/s)" -> [w221]
    tunnel: "Max Ramp Rate - Z Axis (A/s)" -> [w220]
    tunnel: "Operation" -> [w219]
    tunnel: "LI 1" -> [w217]
    tunnel: "HP 1" -> [w216]
    tunnel: "GPIB HP" -> [w215]
    tunnel: "GPIB L 1" -> [w214]
    tunnel: [w213] -> w8
    tunnel: [w212] -> w9
    tunnel: w4 -> [w211]
    tunnel: w3 -> [w210]
    tunnel: w1 -> [w202]
    stop <- w224 continue-if-true
    n85 = stacked-sequence {
      tunnel: w218 -> [w240]
      tunnel: w231 -> [w239]
      tunnel: w230 -> [w238]
      tunnel: w229 -> [w237]
      tunnel: w228 -> [w236]
      tunnel: w227 -> [w235]
      tunnel: [w234] -> w209
      tunnel: [w233] -> w201
      tunnel: [w232] -> w200
      frame #0 {
        # "Read B Field"
        n86 = case shown="1" w240 {
          tunnel: w239 -> [w250 w274]
          tunnel: w238 -> [w249 w273]
          tunnel: w237 -> [w248 w272]
          tunnel: w236 -> [w247 w271]
          tunnel: w235 -> [_ w270]
          tunnel: [w243 w269] -> w233
          tunnel: [w242 w267] -> w232
          tunnel: [w241 w268] -> w234
          tunnel: [_ w266] -> _
          frame #0 {
            n87 = call <userlib>:"Get 2D Field (Cartesian).vi"("Y-Axis Communications Config"=w250, "Z-Axis Communications Config"=w249, "error in"=w248) -> ("All Instruments Responded?"=w244:bool, "Y-Axis Field (kG)"=w246:dbl, "Z-Axis Field (kG)"=w245:dbl, "error out"=w243:T4)  [unwired: 2 in]
            n88 = case shown="1" w247 {
              tunnel: w246 -> [w251 w259]
              tunnel: w245 -> [w252 w260]
              tunnel: w244 -> [w253 w262]
              tunnel: [w252 w258] -> w242
              tunnel: [w251 w257] -> w241
              frame #0 {
                n89 = case shown="True" w253 {
                  tunnel: w251 -> [_ w255]
                  tunnel: w252 -> [_ w254]
                  frame #0 {
                  }
                  frame #1 {
                    n90 = Bundle("Y-Axis Field (kG)"=w255, "Z-Axis Field (kG)"=w254) -> (→"Cartesian Display (kG)":T5)  [unwired: 1 in]
                  }
                }
              }
              frame #1 {
                w261 = 0.1 ("y")
                n91 = Multiply(x=w259, y=w261) -> (x*y=w257:dbl)
                n92 = Multiply(x=w260, y=w261) -> (x*y=w258:dbl)
                n93 = case shown="True" w262 {
                  tunnel: w257 -> [_ w265]
                  tunnel: w258 -> [_ w264]
                  frame #0 {
                  }
                  frame #1 {
                    n94 = Bundle(w265, w264) -> (→"Cartesian Display (T)":cluster{dbl, dbl})  [unwired: 1 in]
                  }
                }
              }
            }
          }
          frame #1 {
            n95 = stacked-sequence {
              tunnel: w274 -> [w285]
              tunnel: w273 -> [w284]
              tunnel: w272 -> [w283]
              tunnel: w271 -> [w282]
              tunnel: w270 -> [w279]
              tunnel: [w277] -> w269
              tunnel: [w275] -> w267
              tunnel: [w276] -> w268
              tunnel: [w275] -> w266
              frame #0 {
                # "Field"
                n96 = call <userlib>:"Get 2D Field (Polar).vi"("Y-Axis Communications Config"=w285, "Z-Axis Communications Config"=w284, "error in"=w283) -> ("All Instruments Responded?"=w278:bool, "Radial (r) Field (kG)"=w281:dbl, "q (radians)"=w280:dbl, "error out"=w277:T4)  [unwired: 2 in]
                n97 = case shown="1" w282 {
                  tunnel: w281 -> [w287 w299]
                  tunnel: w280 -> [w289 w298]
                  tunnel: w279 -> [w288 w297]
                  tunnel: w278 -> [w290 w296]
                  tunnel: [w286 w294] -> w275
                  tunnel: [w286 w295] -> w276
                  frame #0 {
                    n98 = Multiply(x=w289, y=w288) -> (x*y=w286:dbl)
                    n99 = case shown="False" w290 {
                      tunnel: w287 -> [_ w291]
                      tunnel: w286 -> [_ w292]
                      frame #0 {
                      }
                      frame #1 {
                        n100 = Bundle(w292, "Radial (r) Field (kG)"=w291) -> (→"Polar Display (kG)":cluster{dbl, "Radial (r) Field (kG)":dbl})  [unwired: 1 in]
                      }
                    }
                  }
                  frame #1 {
                    n101 = Multiply(x=w299, y=0.1) -> (x*y=w295:dbl)
                    n102 = Multiply(x=w298, y=w297) -> (x*y=w294:dbl)
                    n103 = case shown="True" w296 {
                      tunnel: w295 -> [_ w301]
                      tunnel: w294 -> [_ w302]
                      frame #0 {
                      }
                      frame #1 {
                        n104 = Bundle(w302, w301) -> (→"Polar Display (T)":cluster{dbl, dbl})  [unwired: 1 in]
                      }
                    }
                  }
                }
              }
            }
          }
        }
      }
    }
    n105 = local read "Ramping Control"() -> (w226:u16)
    n106 = Number To Fractional String(number=w209) -> (F-format string=w207:string)  [unwired: 3 in]
    n107 = Number To Fractional String(number=w200) -> (F-format string=w205:string)  [unwired: 3 in]
    n108 = local read "Continue Execution?"() -> (w224:bool)
    n109 = Concatenate Strings("_" ("string"), w207, "_" ("string"), w205, ".txt" ("string")) -> (w203:string)
    n110 = case shown="1" w226 {
      selector: w226 -> [w305 w331 w427 w431 w446]
      tunnel: w213 -> [_ w333 _ w434 w451]
      tunnel: w212 -> [_ w332 _ w433 w450]
      tunnel: [w304 w311 w426 w432 w449] -> w225
      tunnel: [w305 w331 w427 w431 w446] -> w223
      tunnel: w222 -> [_ _ _ w430 w448]
      tunnel: w221 -> [_ _ _ _ w445]
      tunnel: w220 -> [_ _ _ _ w444]
      tunnel: w219 -> [_ w323 _ _ _]
      tunnel: w209 -> [_ w317 _ _ _]
      tunnel: w217 -> [_ w316 _ _ _]
      tunnel: w216 -> [_ w315 _ _ _]
      tunnel: w215 -> [_ w314 _ _ _]
      tunnel: w214 -> [_ w313 _ _ _]
      tunnel: w211 -> [_ w310 _ _ _]
      tunnel: w210 -> [_ w309 _ _ _]
      tunnel: w203 -> [_ w308 _ _ _]
      tunnel: w202 -> [_ w307 _ _ _]
      tunnel: w201 -> [w304 w306 w426 w428 w443]
      frame #0 {
      }
      frame #1 {
        w326 = T8."HOLDING" ("y")
        n111 = local read "Number of lines"() -> (w320:i32)
        n112 = local read "Starting index"() -> (w322:i32)
        n113 = call <userlib>:"Get Ramping Mode.vi"("Communications Config"=w333, "error in"=w306) -> ("Ramping Mode"=w329:T9, "error out"=w330:T4)  [unwired: 1 out]
        n114 = call <userlib>:"Get Ramping Mode.vi"("Communications Config"=w332, "error in"=w330) -> ("Ramping Mode"=w328:T9, "error out"=w312:T4)  [unwired: 1 out]
        n115 = Less?(x=w322, y=w320) -> (x < y?=w321:bool)
        n116 = Equal?(x=w329, y=w326) -> (x = y?=w325:bool)
        n117 = Equal?(x=w328, y=w326) -> (x = y?=w324:bool)
        n118 = Compound Arithmetic op=AND(w325, w324) -> (w327:bool)
        n119 = case shown="True" w327 {
          tunnel: w323 -> [_ w349]
          tunnel: w321 -> [_ w348]
          tunnel: "Wait between \nVectors (ms)" -> [_ w347]
          tunnel: "Wait between \nVectors" -> [_ w346]
          tunnel: w317 -> [_ w345]
          tunnel: w316 -> [_ w344]
          tunnel: w315 -> [_ w343]
          tunnel: w314 -> [_ w342]
          tunnel: w313 -> [_ w341]
          tunnel: w312 -> [w334 w340]
          tunnel: [w334 w339] -> w311
          tunnel: w310 -> [_ w338]
          tunnel: w309 -> [_ w337]
          tunnel: w308 -> [_ w336]
          tunnel: w307 -> [_ w335]
          frame #0 {
          }
          frame #1 {
            n120 = case shown="1" w349 {
              tunnel: w348 -> [_ w366]
              tunnel: w347 -> [_ w365]
              tunnel: w346 -> [_ w364]
              tunnel: w345 -> [_ w363]
              tunnel: w344 -> [_ w362]
              tunnel: w343 -> [_ w361]
              tunnel: w342 -> [_ w360]
              tunnel: w341 -> [_ w359]
              tunnel: w340 -> [w350 w358]
              tunnel: [w350 w357] -> w339
              tunnel: w338 -> [_ w356]
              tunnel: w337 -> [_ w355]
              tunnel: w336 -> [_ w354]
              tunnel: w335 -> [_ w353]
              frame #0 {
                w352 = u16 2 items=["NEXT VECTOR", "RAMPING", "HOLDING", "PAUSE", "ZERO"] ("Ramping Control")
                n121 = local write "STATUS"("Holding at current vector. Set Ramping Mode to NEXT VECTOR to continue." ("STATUS")) -> ()
                n122 = local write "Ramping Control"(w352) -> ()
              }
              frame #1 {
                # "Go to NEXT VECTOR automatically"
                n123 = case shown="True" w366 {
                  tunnel: w365 -> [_ w383]
                  tunnel: w364 -> [_ w382]
                  tunnel: w363 -> [_ w381]
                  tunnel: w362 -> [_ w380]
                  tunnel: w361 -> [_ w379]
                  tunnel: w360 -> [_ w378]
                  tunnel: w359 -> [_ w377]
                  tunnel: w358 -> [w368 w376]
                  tunnel: [w368 w375] -> w357
                  tunnel: w356 -> [_ w374]
                  tunnel: w355 -> [_ w373]
                  tunnel: w354 -> [_ w372]
                  tunnel: w353 -> [_ w371]
                  frame #0 {
                    w370 = u16 2 items=["NEXT VECTOR", "RAMPING", "HOLDING", "PAUSE", "ZERO"] ("Ramping Control")
                    n124 = local write "STATUS"("Holding at current vector. Set Ramping Mode to NEXT VECTOR to continue." ("STATUS")) -> ()
                    n125 = local write "Ramping Control"(w370) -> ()
                    n126 = local write "Continue Execution?"(FALSE) -> ()
                  }
                  frame #1 {
                    n127 = stacked-sequence {
                      tunnel: w383 -> [w396 _]
                      tunnel: w382 -> [w395 _]
                      tunnel: w381 -> [w394 _]
                      tunnel: w380 -> [w393 _]
                      tunnel: w379 -> [w392 _]
                      tunnel: w378 -> [w391 _]
                      tunnel: w377 -> [w390 _]
                      tunnel: w376 -> [w389 _]
                      tunnel: [w388 _] -> w375
                      tunnel: w374 -> [w387 _]
                      tunnel: w373 -> [w386 _]
                      tunnel: w372 -> [w385 _]
                      tunnel: w371 -> [w384 _]
                      frame #0 {
                        n128 = case shown="True" w395 {
                          tunnel: w396 -> [_ w409]
                          tunnel: w394 -> [_ w408]
                          tunnel: w393 -> [_ w407]
                          tunnel: w392 -> [_ w406]
                          tunnel: w391 -> [_ w405]
                          tunnel: w390 -> [_ w401]
                          tunnel: w389 -> [w397 w404]
                          tunnel: [w397 w400] -> w388
                          tunnel: w387 -> [_ w403]
                          tunnel: w386 -> [_ w402]
                          tunnel: w385 -> [_ w399]
                          tunnel: w384 -> [_ w398]
                          frame #0 {
                          }
                          frame #1 {
                            n129 = stacked-sequence {
                              tunnel: w409 -> [w410 _]
                              tunnel: w408 -> [_ _]
                              tunnel: w407 -> [_ w421]
                              tunnel: w406 -> [_ w418]
                              tunnel: w405 -> [_ w419]
                              tunnel: w401 -> [_ _]
                              tunnel: w404 -> [_ w417]
                              tunnel: w403 -> [_ w423]
                              tunnel: w402 -> [_ w422]
                              tunnel: w401 -> [_ w420]
                              tunnel: [_ w417] -> w400
                              tunnel: w399 -> [_ w416]
                              tunnel: w398 -> [_ w415]
                              frame #0 {
                                n130 = Wait (ms)(milliseconds to wait=w410) -> ()  [unwired: 1 out]
                              }
                              frame #1 {
                                n131 = Concatenate Strings(w415, w416) -> (w414:string)
                                n132 = String To Path(string=w414) -> (path=w413:path)
                                n133 = call "K6487 und HP_brassesubvi_2.vi"("GPIB HP"=w419, "HP 1"=w418, "GPIB L 1"=w420, "LI 1"=w421, "Sample name:"=w422, "Notes:"=w423, "Measurement File"=w413) -> ("HP"=→"HP":cluster{dbl[], dbl[]}, "V LI"=→"LI":cluster{dbl[], dbl[]})  [unwired: 3 in]
                              }
                            }
                          }
                        }
                      }
                      frame #1 {
                        w425 = u16 0 items=["NEXT VECTOR", "RAMPING", "HOLDING", "PAUSE", "ZERO"] ("Ramping Control")
                        n134 = local write "Ramping Control"(w425) -> ()
                        n135 = local write "STATUS"("Go to NEXT VECTOR" ("STATUS")) -> ()
                      }
                    }
                  }
                }
              }
            }
          }
        }
      }
      frame #2 {
      }
      frame #3 {
        n136 = Not Equal?(x=w431, y=w430) -> (x != y?=w429:bool)
        n137 = case shown="True" w429 {
          tunnel: w434 -> [_ w442]
          tunnel: w433 -> [_ w441]
          tunnel: [w435 w439] -> w432
          tunnel: w428 -> [w435 w436]
          frame #0 {
          }
          frame #1 {
            w437 = u16 1 items=["RAMP", "PAUSE", "MANUAL UP", "MANUAL DOWN", "ZERO"] ("Ramping Mode")
            n138 = call <userlib>:"Set Ramping Mode.vi"("error in"=w436, "Ramping Mode"=w437, "Communications Config"=w442) -> ("error out"=w440:T4)
            n139 = call <userlib>:"Set Ramping Mode.vi"("error in"=w440, "Ramping Mode"=w437, "Communications Config"=w441) -> ("error out"=w439:T4)
            n140 = local write "STATUS"("All Programmers are PAUSED. Set Ramping Mode to NEXT VECTOR to continue." ("STATUS")) -> ()
          }
        }
      }
      frame #4 {
        n141 = Not Equal?(x=w446, y=w448) -> (x != y?=w447:bool)
        n142 = case shown="False" w447 {
          tunnel: w451 -> [_ w459]
          tunnel: w450 -> [_ w458]
          tunnel: [w452 w454] -> w449
          tunnel: w445 -> [_ w457]
          tunnel: w444 -> [_ w456]
          tunnel: w443 -> [w452 _]
          frame #0 {
          }
          frame #1 {
            w453 = u16 4 items=["RAMP", "PAUSE", "MANUAL UP", "MANUAL DOWN", "ZERO"] ("Ramping Mode")
            n143 = local write "STATUS"("Zeroing vector." ("STATUS")) -> ()
            n144 = call <userlib>:"Set Ramping Mode.vi"("Ramping Mode"=w453, "Communications Config"=w459) -> ("error out"=w462:T4)  [unwired: 1 in]
            n145 = call <userlib>:"Set Ramping Mode.vi"("error in"=w462, "Ramping Mode"=w453, "Communications Config"=w458) -> ("error out"=w455:T4)
            n146 = call <userlib>:"Set Current Ramp Rate.vi"("Communications Config"=w459, "Ramp Rate (A/sec)"=w457, "error in"=w455) -> ("error out"=w460:T4)  [unwired: 2 in]
            n147 = call <userlib>:"Set Current Ramp Rate.vi"("Communications Config"=w458, "Ramp Rate (A/sec)"=w456, "error in"=w460) -> ("error out"=w454:T4)  [unwired: 2 in]
          }
        }
      }
    }
  }
  n148 = local read "Magnetic Field Units"() -> (w58:u16)
  n149 = local read "Coordinate System"() -> (w59:u16)
  n150 = while {
    tunnel: "Starting index" -> [w470]
    tunnel: w12 -> [w476]
    tunnel: w11 -> [w477]
    tunnel: w58 -> [w478]
    tunnel: w59 -> [w479]
    tunnel: w56 -> [w482]
    tunnel: "Max Ramp Rate - Y Axis (A/s)" -> [w466]
    tunnel: "Max Ramp Rate - Z Axis (A/s)" -> [w465]
    tunnel: "Magnitude Limit (kG)" -> [w467]
    tunnel: "User defined Ramp Rate (T/min)" -> [w464]
    tunnel: "User defined Ramp Rate (T/min)" -> [w463]
    i -> [w469]
    stop <- w471 continue-if-true
    n151 = local read "Field Values"() -> (w473:string[][])
    n152 = Add(x=w470, y=w469) -> (x+y=w468:i32)
    n153 = while "Wait for NEXT VECTOR setting by operator." {
      tunnel: [w486] -> w481
      tunnel: w482 -> [w486]
      stop <- w487 continue-if-true
      w485 = u16 0 items=["NEXT VECTOR", "RAMPING", "HOLDING", "PAUSE", "ZERO"] ("Ramping Control")
      n154 = local read "Ramping Control"() -> (w488:u16)
      n155 = Not Equal?(x=w485, y=w488) -> (x != y?=w487:bool)
    }
    n156 = stacked-sequence {
      tunnel: w468 -> [w490 _ w496 _]
      frame #0 {
        (unwired) -2
        n157 = Subtract(x=w490, y=2) -> (x-y=w493:i32)
        n158 = Bundle(w493, -2) -> (w491:cluster{i32, i32})  [unwired: 1 in]
        n159 = property on="Field Values" class="Tbl (strict)"("Active Cell:Active Cell"=w491) -> ()  [unwired: 2 in, 2 out]
      }
      frame #1 {
        n160 = local read "Normal color"() -> (w494:u32)
        n161 = property on="Field Values" class="Tbl (strict)"("Active Cell:Cell Background Color"=w494) -> ()  [unwired: 2 in, 2 out]
      }
      frame #2 {
        n162 = Decrement(x=w496) -> (x-1=w495:i32)
        n163 = Bundle(w495, -2) -> (w498:cluster{i32, i32})  [unwired: 1 in]
        n164 = property on="Field Values" class="Tbl (strict)"("Active Cell:Active Cell"=w498) -> ()  [unwired: 2 in, 2 out]
      }
      frame #3 {
        n165 = property on="Field Values" class="Tbl (strict)"("Active Cell:Cell Background Color"="Highlight color") -> ()  [unwired: 2 in, 2 out]
      }
    }
    n166 = Index Array(array=w473, index (row)=w468) -> (element=w480:string[])  [unwired: 1 in]
    "fieldvalues" <- w480
    n167 = local write "Starting index"(w468) -> ()
    n168 = Add(x=1, y=w468) -> (x+y=w483:i32)
    n169 = Number To Decimal String(number=w483) -> (decimal integer string=w472:string)  [unwired: 1 in]
    n170 = stacked-sequence {
      tunnel: [_ w524] -> w474
      tunnel: [_ w523] -> w475
      tunnel: w481 -> [_ w519]
      tunnel: w480 -> [_ w518]
      tunnel: w479 -> [_ w517]
      tunnel: w478 -> [_ w516]
      tunnel: w477 -> [_ w515]
      tunnel: w476 -> [_ w514]
      tunnel: w472 -> [_ w513]
      tunnel: w467 -> [_ w511]
      tunnel: w466 -> [_ w510]
      tunnel: w465 -> [_ w505]
      tunnel: w464 -> [_ w509]
      tunnel: w463 -> [_ w508]
      frame #0 {
        w503 = u16 1 items=["NEXT VECTOR", "RAMPING", "HOLDING", "PAUSE", "ZERO"] ("Ramping Control")
        n171 = local write "Ramping Control"(w503) -> ()
      }
      frame #1 {
        n172 = call <userlib>:"Set 2D Next Vector_entwurf.vi"("Coordinate System"=w517, "Magnetic Field Units"=w516, 3:"User defined Ramp Rate (T/min)"=w508, "Magnitude Limit (kG)"=w511, "Y-Axis Communications Config"=w515, "Input Vector"=w518, "Z-Axis Communications Config"=w514, 10:"User defined Ramp Rate (T/min)"=w509, "Max Ramp Rate - Y Axis (A/s)"=w510, "error in"=w519, "Max Ramp Rate - Z Axis (A/s)"=w505) -> ("Y-Axis Ramp Rate (T/min)"=→"Current Ramp Rate Y (T/min)":dbl, "Within Limits?"=w524:bool, "Ramp Rate along Vector (T/min)"=→"Ramp Rate along Vector (T/min)":dbl, "Z-Axis Ramp Rate (T/min)"=→"Current Ramp Rate Z (T/min)":dbl, "All Instruments Responded?"=w523:bool, "error out"=w512:T4)  [unwired: 3 in]
        n173 = Concatenate Strings("Ramping to field vector " ("STATUS"), w513, "..." ("STATUS")) -> (w520:string)
        n174 = local write "error in"(w512) -> ()
        n175 = local write "STATUS"(w520) -> ()
      }
    }
    n176 = case shown="True" w474 {
      tunnel: w475 -> [_ w501]
      frame #0 {
        n177 = local write "STATUS"("Vector magnitude limt or maximum coil current exceeded. Vector ignored. VI halted." ("STATUS")) -> ()
      }
      frame #1 {
        n178 = case shown="True" w501 {
          frame #0 {
            n179 = local write "STATUS"("Not all programmers responded. VI halted." ("STATUS")) -> ()
          }
          frame #1 {
          }
        }
      }
    }
    n180 = Compound Arithmetic op=AND(w475, w474) -> (w471:bool)
    n181 = local write "Continue Execution?"(w471) -> ()
  }
  n182 = case shown="True" "go to zero at end of measurement" {
    tunnel: [w525 w529] -> w10
    tunnel: w9 -> [_ w528]
    tunnel: w8 -> [_ w527]
    tunnel: w7 -> [w525 w526]
    frame #0 {
      # "go to zero"
    }
    frame #1 {
      n183 = stacked-sequence {
        tunnel: w527 -> [w546]
        tunnel: w528 -> [w547]
        tunnel: w526 -> [w537]
        tunnel: [w536] -> _
        frame #0 {
          w541 = u16 0 items=["kG", "Tesla"] ("Magnetic Field Units")
          w542 = u16 0 items=["Cartesian", "Polar"] ("Coordinate System")
          n184 = Build Array("0", "0") -> (w543:string[])
          n185 = call <userlib>:"Set 2D Next Vector_entwurf.vi"("Coordinate System"=w542, "Magnetic Field Units"=w541, "Magnitude Limit (kG)"=45.0, "Y-Axis Communications Config"=w546, "Input Vector"=w543, "Z-Axis Communications Config"=w547, "User defined Ramp Rate (T/min)"=FALSE, "Max Ramp Rate - Y Axis (A/s)"=0.05, "error in"=w537, "Max Ramp Rate - Z Axis (A/s)"=0.15) -> ("error out"=w536:T4)  [unwired: 4 in, 5 out]
        }
      }
      n186 = local read "Magnetic Field Units"() -> (w531:u16)
      n187 = local read "Coordinate System"() -> (w532:u16)
      n188 = Divide(x=180.0, y=3.141592653589793) -> (x/y=w530:dbl)
      n189 = while {
        tunnel: w530 -> [w556]
        tunnel: w531 -> [w557]
        tunnel: w528 -> [w553]
        tunnel: w527 -> [w554]
        tunnel: [w555] -> _
        tunnel: w532 -> [w555]
        tunnel: [w551] -> w529
        tunnel: w526 -> [w550]
        stop <- w552 stop-if-true
        n190 = stacked-sequence {
          tunnel: w555 -> [w602]
          tunnel: w554 -> [w601]
          tunnel: w553 -> [w600]
          tunnel: w557 -> [w599]
          tunnel: w556 -> [w598]
          tunnel: w550 -> [w597]
          tunnel: [w596] -> w548
          frame #0 {
            # "Read B Field"
            n191 = case shown="1" w602 {
              tunnel: w601 -> [w612 w634]
              tunnel: w600 -> [w611 w633]
              tunnel: w599 -> [w610 w632]
              tunnel: w598 -> [_ w631]
              tunnel: [w606 w630] -> w596
              tunnel: [w605 w628] -> _
              tunnel: [w604 w629] -> _
              tunnel: w597 -> [w603 _]
              frame #0 {
                n192 = call <userlib>:"Get 2D Field (Cartesian).vi"("Y-Axis Communications Config"=w612, "Z-Axis Communications Config"=w611, "error in"=w603) -> ("All Instruments Responded?"=w607:bool, "Y-Axis Field (kG)"=w609:dbl, "Z-Axis Field (kG)"=w608:dbl, "error out"=w606:T4)  [unwired: 2 in]
                n193 = case shown="1" w610 {
                  tunnel: w609 -> [w613 w621]
                  tunnel: w608 -> [w614 w622]
                  tunnel: w607 -> [w615 w624]
                  tunnel: [w614 w620] -> w605
                  tunnel: [w613 w619] -> w604
                  frame #0 {
                    n194 = case shown="False" w615 {
                      tunnel: w613 -> [_ w618]
                      tunnel: w614 -> [_ w617]
                      frame #0 {
                      }
                      frame #1 {
                        n195 = Bundle("Y-Axis Field (kG)"=w618, "Z-Axis Field (kG)"=w617) -> (w616:T5)  [unwired: 1 in]
                        n196 = local write "Cartesian Display (kG)"(w616) -> ()
                      }
                    }
                  }
                  frame #1 {
                    w623 = 0.1 ("y")
                    n197 = Multiply(x=w621, y=w623) -> (x*y=w619:dbl)
                    n198 = Multiply(x=w622, y=w623) -> (x*y=w620:dbl)
                    n199 = case shown="True" w624 {
                      tunnel: w619 -> [_ w627]
                      tunnel: w620 -> [_ w626]
                      frame #0 {
                      }
                      frame #1 {
                        n200 = Bundle(w627, w626) -> (w625:cluster{dbl, dbl})  [unwired: 1 in]
                        n201 = local write "Cartesian Display (T)"(w625) -> ()
                      }
                    }
                  }
                }
              }
              frame #1 {
                n202 = stacked-sequence {
                  tunnel: w634 -> [w644]
                  tunnel: w633 -> [w643]
                  tunnel: w632 -> [w642]
                  tunnel: w631 -> [w639]
                  tunnel: [w637] -> w630
                  tunnel: [w636] -> w628
                  tunnel: [w635] -> w629
                  frame #0 {
                    # "Field"
                    n203 = call <userlib>:"Get 2D Field (Polar).vi"("Y-Axis Communications Config"=w644, "Z-Axis Communications Config"=w643) -> ("All Instruments Responded?"=w638:bool, "Radial (r) Field (kG)"=w641:dbl, "q (radians)"=w640:dbl, "error out"=w637:T4)  [unwired: 3 in]
                    n204 = case shown="1" w642 {
                      tunnel: w641 -> [w646 w658]
                      tunnel: w640 -> [w648 w657]
                      tunnel: w639 -> [w647 w656]
                      tunnel: w638 -> [w649 w655]
                      tunnel: [w646 w653] -> w636
                      tunnel: [w645 w654] -> w635
                      frame #0 {
                        n205 = Multiply(x=w648, y=w647) -> (x*y=w645:dbl)
                        n206 = case shown="True" w649 {
                          tunnel: w646 -> [_ w651]
                          tunnel: w645 -> [_ w652]
                          frame #0 {
                          }
                          frame #1 {
                            n207 = Bundle(w652, "Radial (r) Field (kG)"=w651) -> (w650:cluster{dbl, "Radial (r) Field (kG)":dbl})  [unwired: 1 in]
                            n208 = local write "Polar Display (kG)"(w650) -> ()
                          }
                        }
                      }
                      frame #1 {
                        n209 = Multiply(x=w658, y=0.1) -> (x*y=w654:dbl)
                        n210 = Multiply(x=w657, y=w656) -> (x*y=w653:dbl)
                        n211 = case shown="True" w655 {
                          tunnel: w654 -> [_ w661]
                          tunnel: w653 -> [_ w662]
                          frame #0 {
                          }
                          frame #1 {
                            n212 = Bundle(w662, w661) -> (w660:cluster{dbl, dbl})  [unwired: 1 in]
                            n213 = local write "Polar Display (T)"(w660) -> ()
                          }
                        }
                      }
                    }
                  }
                }
              }
            }
          }
        }
        n214 = local read "PID Off"() -> (w549:bool)
        n215 = stacked-sequence {
          seq-local: [w559 _ _ _] -> [_ w570 w581 w591]
          seq-local: [w558 _ _ _] -> [_ _ w580 _]
          tunnel: w554 -> [w568 _ w583 _]
          tunnel: w553 -> [w567 _ w582 _]
          tunnel: w548 -> [w566 _ _ _]
          tunnel: [w559 _ _ _] -> w552
          tunnel: [_ _ w579 _] -> w551
          tunnel: w549 -> [_ w569 _ _]
          frame #0 {
            w562 = T8."HOLDING" ("y")
            n216 = call <userlib>:"Get Ramping Mode.vi"("Communications Config"=w568, "error in"=w566) -> ("Ramping Mode"=w564:T9, "error out"=w565:T4)  [unwired: 1 out]
            n217 = call <userlib>:"Get Ramping Mode.vi"("Communications Config"=w567, "error in"=w565) -> ("Ramping Mode"=w563:T9, "error out"=w558:T4)  [unwired: 1 out]
            n218 = Equal?(x=w563, y=w562) -> (x = y?=w561:bool)
            n219 = Equal?(x=w564, y=w562) -> (x = y?=w560:bool)
            n220 = And(x=w560, y=w561) -> (x .and. y?=w559:bool)
          }
          frame #1 {
            n221 = case shown="True" w570 {
              tunnel: w569 -> [_ w571]
              frame #0 {
              }
              frame #1 {
                n222 = case shown="True" w571 {
                  frame #0 {
                  }
                  frame #1 {
                    n223 = flat-sequence {
                      frame #0 {
                        n224 = call "SIM960Poff.vi"("off/on (0/1)"="0", "Port Num- PID"="1", "GPIB-Adress"="2") -> ()  [unwired: 9 in]
                      }
                      frame #1 {
                        n225 = call "SIM960Poff.vi"("off/on (0/1)"="0", "Port Num- PID"="3", "GPIB-Adress"="2") -> ()  [unwired: 9 in]
                      }
                    }
                  }
                }
                n226 = Wait (ms)(milliseconds to wait=u32 40000) -> ()  [unwired: 1 out]
              }
            }
          }
          frame #2 {
            n227 = case shown="True" w581 {
              tunnel: w583 -> [_ w590]
              tunnel: w582 -> [_ w589]
              tunnel: [w584 w586] -> w579
              tunnel: w580 -> [w584 w585]
              frame #0 {
              }
              frame #1 {
                w587 = u16 1 items=["RAMP", "PAUSE", "MANUAL UP", "MANUAL DOWN", "ZERO"] ("Ramping Mode")
                n228 = call <userlib>:"Set Ramping Mode.vi"("error in"=w585, "Ramping Mode"=w587, "Communications Config"=w590) -> ("error out"=w588:T4)
                n229 = call <userlib>:"Set Ramping Mode.vi"("error in"=w588, "Ramping Mode"=w587, "Communications Config"=w589) -> ("error out"=w586:T4)
              }
            }
          }
          frame #3 {
            n230 = case shown="True" w591 {
              frame #0 {
              }
              frame #1 {
                n231 = call <userlib>:"430_TCP_PSoff.vi"("IP Address"="111.111.111.2", "Switch Heater Control"=FALSE) -> ()  [unwired: 5 in, 2 out]
                n232 = call <userlib>:"430_TCP_PSoff.vi"("IP Address"="111.111.111.1", "Switch Heater Control"=FALSE) -> ()  [unwired: 5 in, 2 out]
              }
            }
          }
        }
      }
    }
  }
  n233 = Unbundle By Name(w12) -> ("Active Comm Interface"=w39:u16, "connection ID"=w38:refnum<k5>, "Serial Port"=w37:refnum<visa-resource-name>)
  n234 = Unbundle By Name(w11) -> ("Active Comm Interface"=w40:u16, "connection ID"=w36:refnum<k5>, "Serial Port"=w35:refnum<visa-resource-name>)
  n235 = case shown="0, Default" w40 {
    tunnel: w36 -> [w665 _ _]
    tunnel: [w664 w668 w669] -> w41
    tunnel: w35 -> [_ w667 _]
    tunnel: w10 -> [w663 w666 w669]
    frame #0 {
      n236 = call <userlib>:"430_TCP_Close.vi"("error in (no error)"=w663, "connection ID"=w665) -> ("error out"=w664:errorcluster)  [unwired: 1 out]
    }
    frame #1 {
      n237 = call <userlib>:"430_RS232_Close.vi"("error in (no error)"=w666, "VISA resource name"=w667) -> ("error out"=w668:errorcluster)  [unwired: 1 in]
    }
    frame #2 {
    }
  }
  n238 = case shown="0, Default" w39 {
    tunnel: w38 -> [w672 _ _]
    tunnel: w41 -> [w671 w675 w676]
    tunnel: [w670 w674 w676] -> w34
    tunnel: w37 -> [_ w673 _]
    frame #0 {
      n239 = call <userlib>:"430_TCP_Close.vi"("error in (no error)"=w671, "connection ID"=w672) -> ("error out"=w670:errorcluster)  [unwired: 1 out]
    }
    frame #1 {
      n240 = call <userlib>:"430_RS232_Close.vi"("error in (no error)"=w675, "VISA resource name"=w673) -> ("error out"=w674:errorcluster)  [unwired: 1 in]
    }
    frame #2 {
    }
  }
  "error out" <- w34
